vi "Initialize Async Reference.vi"(8 "error in (no error)":errorcluster, 11 "Test Number and Bin Generator in":refnum<class "Test Number and Bin Generator.lvclass">=refnum) -> (0 "error out":errorcluster, 3 "Test Number and Bin Generator out":refnum<class "Test Number and Bin Generator.lvclass">)   [LabVIEW 2018, in "Test Number and Bin Generator.lvlib" / "Test Number and Bin Generator.lvclass"]
uses:
  Test Number and Bin Generator.lvclass
  Test Number and Bin Generator.lvclass/Test Number and Bin Generator.ctl
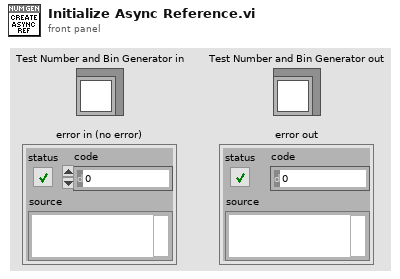
[diagram p1: front panel]
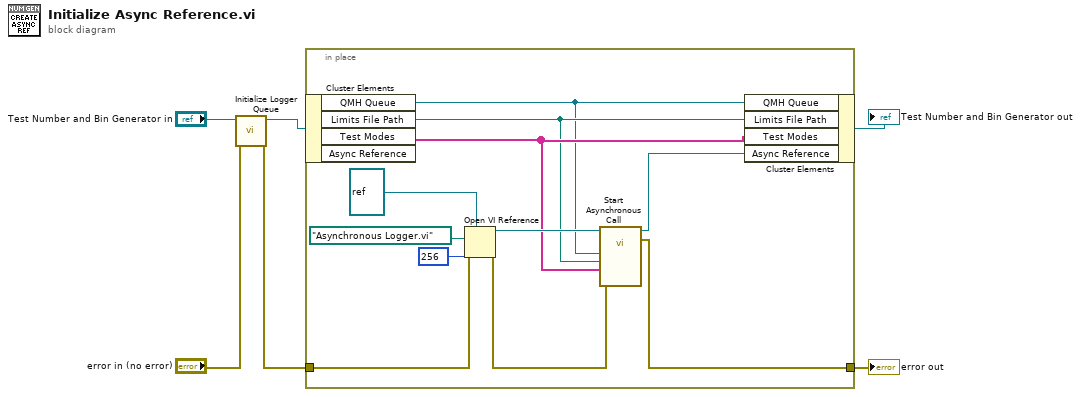
[diagram p0: block diagram]
diagram:
  n1 = call "Initialize Logger Queue.vi"("error in (no error)"="error in (no error)", "Test Number and Bin Generator in"="Test Number and Bin Generator in") -> ("error out"=w4:errorcluster, "Test Number and Bin Generator out"=w2:refnum<class "Test Number and Bin Generator.lvclass">)  [unwired: 8 in]
  n2 = in-place {
    in-place-border: [w7] -> w5
    in-place-border: w4 -> [w13]
    n3 = in-place-cluster #1(w2) -> ("QMH Queue"=w10:refnum<queue>, "Limits File Path"=w11:path, "Test Modes"=w12:string[])  [unwired: 1 out]
    n4 = Open VI Reference(type specifier VI Refnum (for type only)=refnum<vi> refnum ("Async Reference"), vi path=path "Asynchronous Logger.vi", options=256, error in (no error)=w13) -> (vi reference=w15:refnum<vi>, error out=w14:errorcluster)  [unwired: 2 in]
    n5 = call-by-ref "Start Asynchronous Call"(reference=w15, error in=w14, "Test Modes"=w12, "Limits File Path"=w11, "QMH Queue"=w10) -> (reference out=w8:refnum<vi>, error out=w7:errorcluster)  [unwired: 8 in, 1 out]
    n6 = in-place-cluster #1("QMH Queue"=w10, "Limits File Path"=w11, "Test Modes"=w12, "Async Reference"=w8) -> (→"Test Number and Bin Generator out":refnum<class "Test Number and Bin Generator.lvclass">)
  }
  "error out" <- w5
